vi "serial_config_panel.vi"(7 "Error In":errorcluster, 10 "Serial Settings":T1={"baud rate"=9600, "data bits"=8, "parity"=enum."None", "stop bits"=10, "flow control"=0, "IsConfigured"=FALSE} {"flow control" items=["None"=0, "XON/XOFF"=1, "RTS/CTS"=2, "DTR/DSR"=4]; "stop bits" items=["1.0"=10, "1.5"=15, "2.0"=20]; "data bits" min=5 max=8 step=1; "baud rate" items=["75"=75, "110"=110, "134"=134, "150"=150, "300"=300, "600"=600, "1200"=1200, "1800"=1800, "2400"=2400, "4800"=4800, "7200"=7200, "9600"=9600, "14400"=14400, "19200"=19200, "28800"=28800, "38400"=38400, "56000"=56000, "57600"=57600, "115200"=115200, "128000"=128000, "230400"=230400]}) -> (0 "Error Out":errorcluster, 3 "Serial Settings 2":T1={"baud rate"=9600, "data bits"=8, "parity"=enum."None", "stop bits"=10, "flow control"=0, "IsConfigured"=FALSE} {"flow control" items=["None"=0, "XON/XOFF"=1, "RTS/CTS"=2, "DTR/DSR"=4]; "stop bits" items=["1.0"=10, "1.5"=15, "2.0"=20]; "data bits" min=5 max=8 step=1; "baud rate" items=["75"=75, "110"=110, "134"=134, "150"=150, "300"=300, "600"=600, "1200"=1200, "1800"=1800, "2400"=2400, "4800"=4800, "7200"=7200, "9600"=9600, "14400"=14400, "19200"=19200, "28800"=28800, "38400"=38400, "56000"=56000, "57600"=57600, "115200"=115200, "128000"=128000, "230400"=230400]})   [LabVIEW 2017]
uses:
  serial_setting_1.ctl
panel:
  in  "Default":bool
  in  "Cancel Button":bool
  in  "OK Button":bool
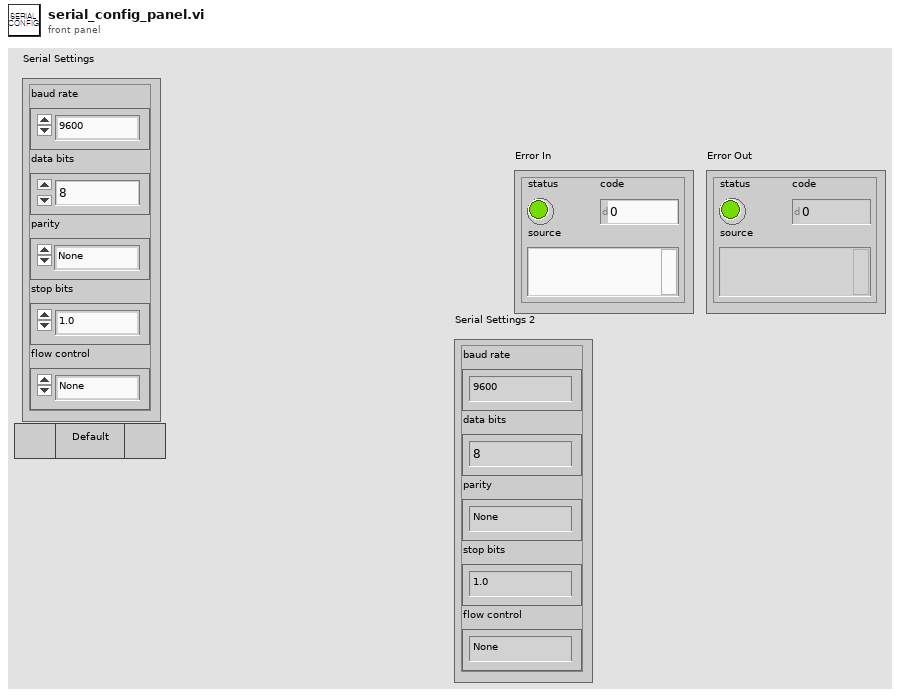
[diagram p1: front panel]
types:
  T1 = typedef "serial_setting_1.ctl" = cluster{"baud rate":u32, "data bits":u16, "parity":enum16{"None", "Odd", "Even", "Mark", "Space"}, "stop bits":u16, "flow control":u16, "IsConfigured":bool}
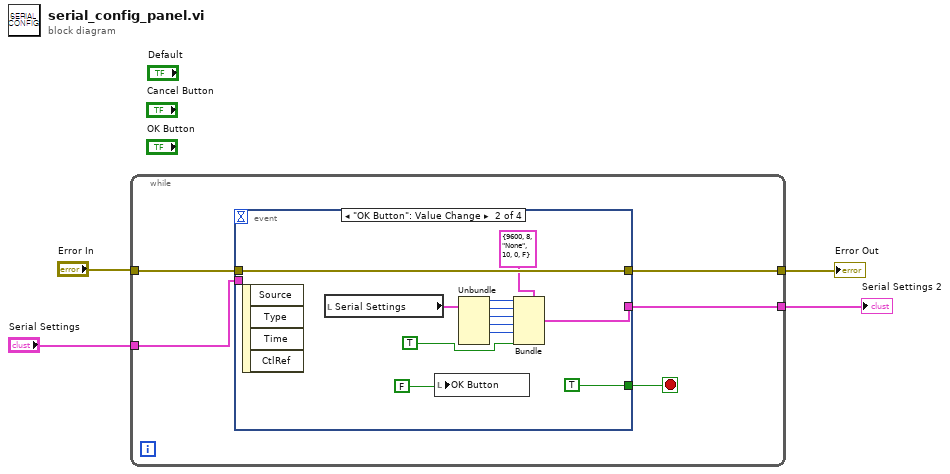
[diagram p0: block diagram]
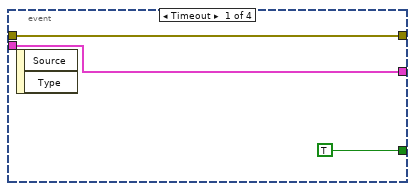
[diagram p2: hidden frame]
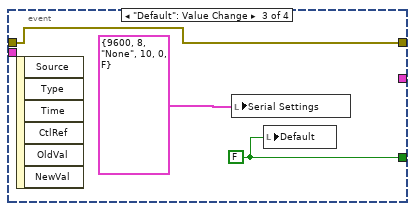
[diagram p3: hidden frame]
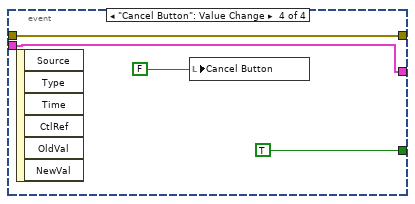
[diagram p4: hidden frame]
diagram:
  n1 = while {
    tunnel: "Error In" -> [w8]
    tunnel: [w7] -> w3
    tunnel: [w6] -> w2
    tunnel: "Serial Settings" -> [w5]
    stop <- w9 stop-if-true
    n2 = event shown="[1] \"OK Button\": Value Change" {
      selector: _ -> [_ _ _ _]
      dyn-events: _ -> [_ _ _ _]
      timeout: _ -> [_ _ _ _]
      tunnel: [TRUE TRUE w27 TRUE] -> w9
      tunnel: [w11 w22 w26 w29] -> w7
      tunnel: w8 -> [w11 w22 w26 w29]
      tunnel: [w10 w20 _ w28] -> w6
      tunnel: w5 -> [w10 _ _ w28]
      event Timeout {
        n3 = event-data() -> ()  [unwired: 1 in, 2 out]
      }
      event "OK Button": Value Change {
        n4 = event-data() -> ()  [unwired: 1 in, 4 out]
        n5 = local read "Serial Settings"() -> (w21:T1)
        n6 = local write "OK Button"(FALSE) -> ()
        n7 = Unbundle(w21) -> ("baud rate"=w19:u32, "data bits"=w18:u16, "parity"=w17:enum16{"None", "Odd", "Even", "Mark", "Space"}, "stop bits"=w16:u16, "flow control"=w15:u16)  [unwired: 1 out]
        n8 = Bundle(cluster=T1 {"baud rate"=9600, "data bits"=8, "parity"=enum."None", "stop bits"=10, "flow control"=0, "IsConfigured"=FALSE} ("Serial Settings"), "baud rate"=w19, "data bits"=w18, "parity"=w17, "stop bits"=w16, "flow control"=w15, "IsConfigured"=TRUE) -> (w20:T1)
      }
      event "Default": Value Change {
        w27 = FALSE
        n9 = event-data() -> ()  [unwired: 1 in, 6 out]
        n10 = local write "Serial Settings"(T1 {"baud rate"=9600, "data bits"=8, "parity"=enum."None", "stop bits"=10, "flow control"=0, "IsConfigured"=FALSE} ("Serial Settings")) -> ()
        n11 = local write "Default"(w27) -> ()
      }
      event "Cancel Button": Value Change {
        n12 = event-data() -> ()  [unwired: 1 in, 6 out]
        n13 = local write "Cancel Button"(FALSE) -> ()
      }
    }
  }
  "Error Out" <- w3
  "Serial Settings 2" <- w2
